vi "globalsettings.vi"() -> ()   [LabVIEW 2012]
panel:
  out "DO":T1
  out "COEFFICIENT":T2
  out "Tangent":T3
  out "BLUE":T4
  out "RED":T4
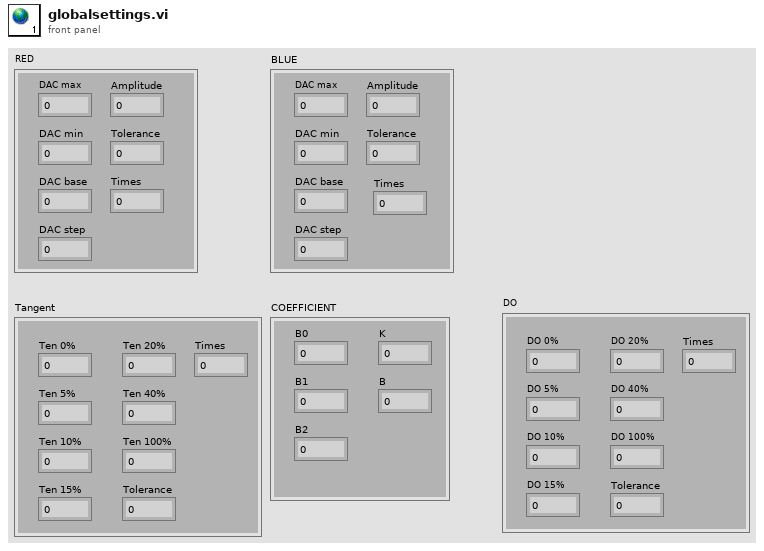
[diagram p1: front panel]
types:
  T1 = cluster{"DO 0%":dbl, "DO 5%":dbl, "DO 10%":dbl, "DO 20%":dbl, "Tolerance":dbl, "DO 15%":dbl, "DO 40%":dbl, "DO 100%":dbl, "Times":dbl}
  T2 = cluster{"B0":dbl, "B1":dbl, "K":dbl, "B":dbl, "B2":dbl}
  T3 = cluster{"Ten 0%":dbl, "Ten 5%":dbl, "Ten 10%":dbl, "Ten 20%":dbl, "Tolerance":dbl, "Ten 15%":dbl, "Ten 40%":dbl, "Ten 100%":dbl, "Times":dbl}
  T4 = cluster{"DAC max":dbl, "DAC min":dbl, "DAC base":dbl, "DAC step":dbl, "Amplitude":dbl, "Tolerance":dbl, "Times":dbl}
diagram:
